vi "Subvi photon counter.vi"(5 "DI channel":refnum<k21>="Connector0/DIO1", 12 "Photon counter input selector":u8) -> (1 "PMT mon":bool, 2 "PMT edge change mon":bool, 3 "Gated pixel clock change mon":bool, 6 "Count":u8)   [LabVIEW 2017]
uses:
  <vilib>/rvi/eio/common/nirviEmuTemplateMethod_errors.vi
  GV PMT sim.vi
  GV gated pixel clock change.vi
  <vilib>/eio/EIONode/EIONode.xnode
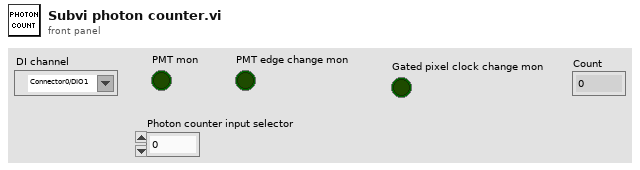
[diagram p1: front panel]
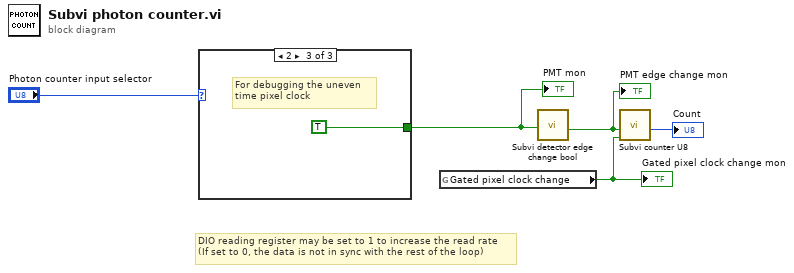
[diagram p0: block diagram]
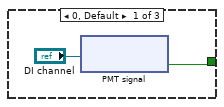
[diagram p2: hidden frame]
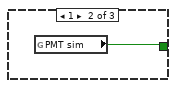
[diagram p3: hidden frame]
diagram:
  # "DIO reading register may be set to 1 to increase the read rate\n(If set to 0, the data is not in sync with the rest of the loop)"
  n1 = case shown="2" "Photon counter input selector" {
    tunnel: [w6 w8 TRUE] -> w1
    frame 0, Default {
      n2 = xnode "PMT signal"("FPGA I/O In"="DI channel") -> ("I/O Item"=w6:bool)  [unwired: 1 out]
    }
    frame 1 {
      n3 = global read "GV PMT sim.vi" "PMT sim"() -> (w8:bool)
    }
    frame 2 {
      # "For debugging the uneven\ntime pixel clock"
    }
  }
  "PMT mon" <- w1
  n4 = global read "GV gated pixel clock change.vi" "Gated pixel clock change"() -> (w4:bool)
  "Gated pixel clock change mon" <- w4
  n5 = call "Subvi detector edge change bool.vi"("Input"=w1) -> ("Output"=w5:bool)  [unwired: 8 in]
  "PMT edge change mon" <- w5
  n6 = call "Subvi counter U8.vi"("Reset"=w4, "+1"=w5) -> ("Count"=→"Count":u8)  [unwired: 9 in]
